vi "PasteCSV example.vi"() -> ()   [LabVIEW 2018]
panel:
  in  "U8":u8[][](array[numeric])
  in  "Float":dbl[][](array[numeric])
  in  "Array String":string[][](array[string])
  in  "Table Control":string[][](table)
  in  "Multicolumn Listbox":i32(listbox)
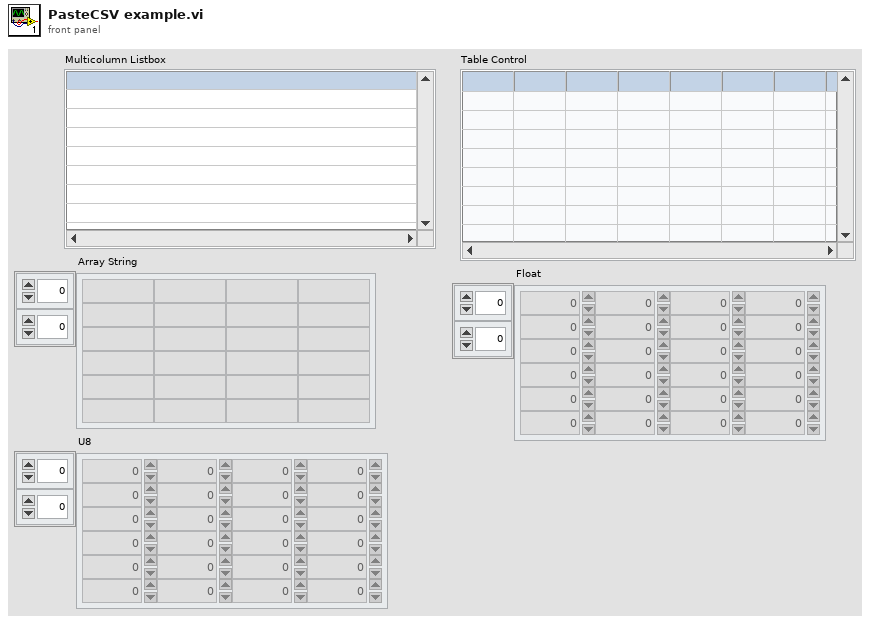
[diagram p1: front panel]
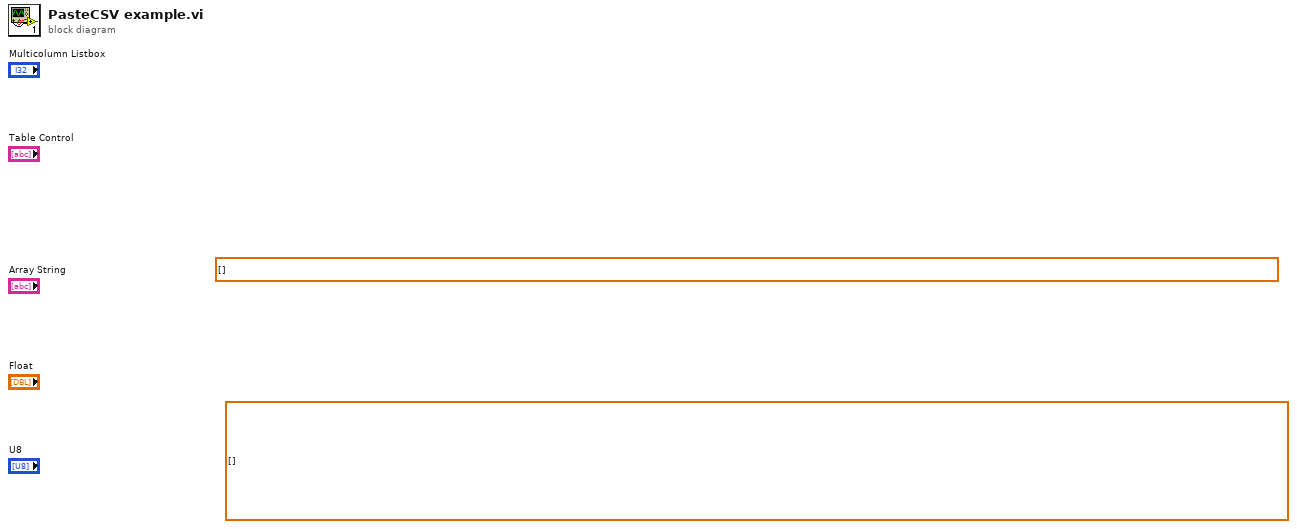
[diagram p0: block diagram]
diagram:
  (unwired) dbl[] [] ("Float")
  (unwired) dbl[][] [] ("Float")
